vi "SRT-2014-Controls-Basic.vi"() -> ()   [LabVIEW 2013]
uses:
  <vilib>/DAQmx/write.llb/DAQmx Write (Digital Bool 1Line 1Point).vi
  <vilib>/DAQmx/miscellaneous.llb/DAQmx Fill In Error Info.vi
panel:
  out "Ignition":bool
  in  "Ignite":bool
  out "NO2 Venting":bool
  out "NO2 Filling":bool
  in  "Emergency Stop":bool
  in  "Disconnected":bool
  in  "Done W/ NO2":bool
  in  "NO2 QD":bool
  in  "NO2 Vent":bool
  in  "NO2 Fill":bool
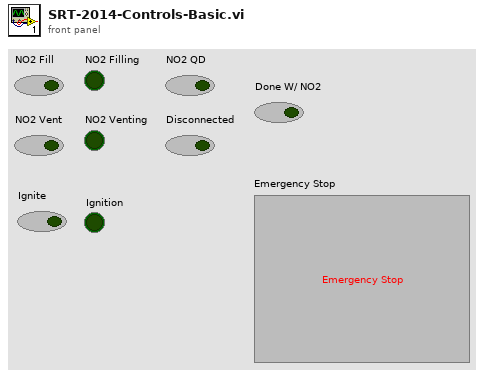
[diagram p1: front panel]
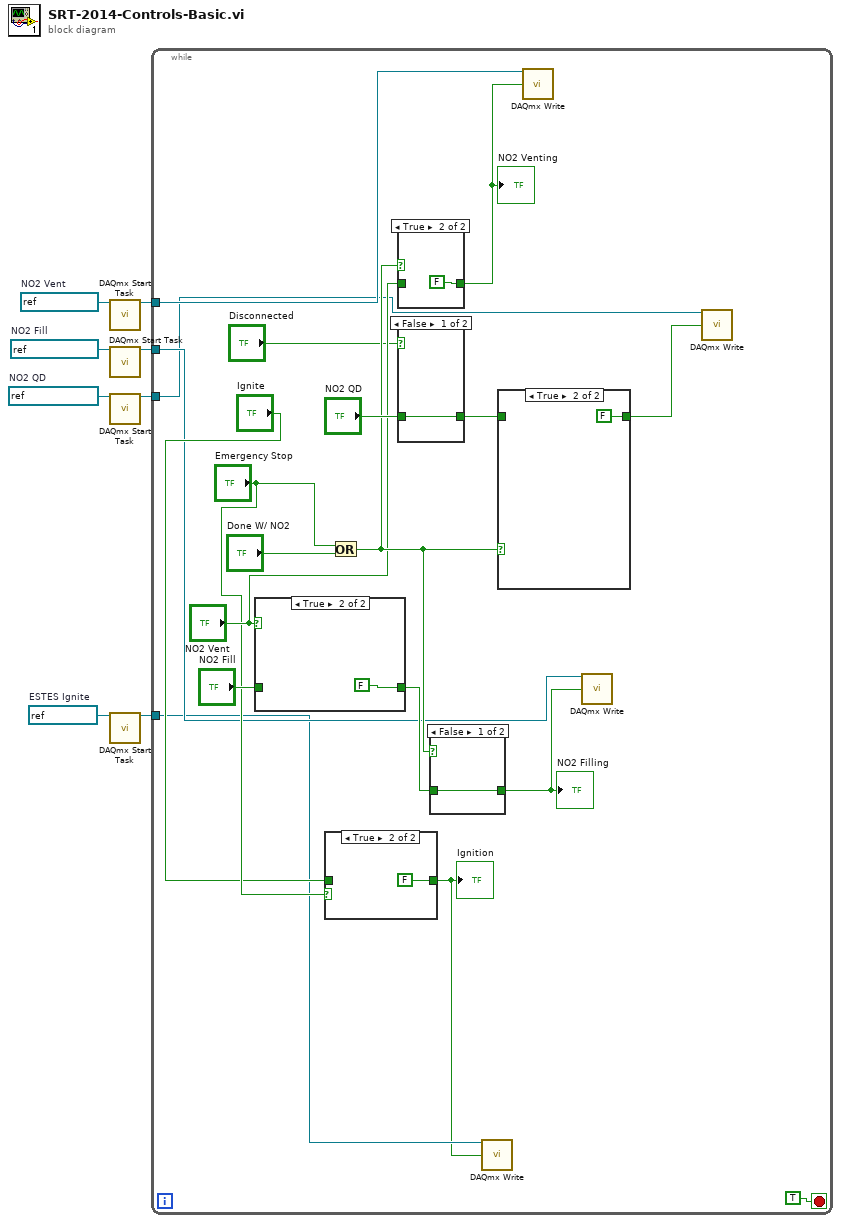
[diagram p0: block diagram]
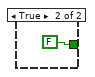
[diagram p4: hidden frame]
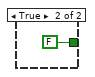
[diagram p6: hidden frame]
diagram:
  w2 = refnum<k21> "2_3"  # ESTES Ignite
  w6 = refnum<k21> "1_0"  # NO2 Fill
  w4 = refnum<k21> "1_2"  # NO2 QD
  w8 = refnum<k21> "1_1"  # NO2 Vent
  n1 = call <vilib>:"DAQmx Start Task.vi"("task/channels in"=w8) -> ("task out"=w7:refnum<k21>)  [unwired: 13 in, 1 out]
  n2 = call <vilib>:"DAQmx Start Task.vi"("task/channels in"=w6) -> ("task out"=w5:refnum<k21>)  [unwired: 13 in, 1 out]
  n3 = call <vilib>:"DAQmx Start Task.vi"("task/channels in"=w4) -> ("task out"=w3:refnum<k21>)  [unwired: 13 in, 1 out]
  n4 = call <vilib>:"DAQmx Start Task.vi"("task/channels in"=w2) -> ("task out"=w1:refnum<k21>)  [unwired: 13 in, 1 out]
  n5 = while {
    tunnel: w7 -> [w16]
    tunnel: w5 -> [w14]
    tunnel: w3 -> [w12]
    tunnel: w1 -> [w10]
    stop <- TRUE stop-if-true
    n6 = case shown="True" "NO2 Vent" {
      tunnel: "NO2 Fill" -> [w38 _]
      tunnel: [w38 FALSE] -> w25
      frame False {
      }
      frame True {
      }
    }
    n7 = case shown="True" "Emergency Stop" {
      tunnel: [w28 FALSE] -> w9
      tunnel: "Ignite" -> [w28 _]
      frame False {
      }
      frame True {
      }
    }
    "Ignition" <- w9
    n8 = Or(x="Emergency Stop", y="Done W/ NO2") -> (x .or. y?=w22:bool)
    n9 = case shown="True" w22 {
      tunnel: [w34 FALSE] -> w15
      tunnel: "NO2 Vent" -> [w34 _]
      frame False {
      }
      frame True {
      }
    }
    "NO2 Venting" <- w15
    n10 = case shown="False" "Disconnected" {
      tunnel: "NO2 QD" -> [w36 _]
      tunnel: [w36 FALSE] -> w24
      frame False {
      }
      frame True {
      }
    }
    n11 = case shown="False" w22 {
      tunnel: w25 -> [w32 _]
      tunnel: [w32 FALSE] -> w13
      frame False {
      }
      frame True {
      }
    }
    "NO2 Filling" <- w13
    n12 = call-poly <vilib>:"DAQmx Write.vi"("task/channels in"=w10, "data"=w9) -> ()  [unwired: 11 in, 3 out]
    n13 = case shown="True" w22 {
      tunnel: w24 -> [w30 _]
      tunnel: [w30 FALSE] -> w11
      frame False {
      }
      frame True {
      }
    }
    n14 = call-poly <vilib>:"DAQmx Write.vi"("task/channels in"=w16, "data"=w15) -> ()  [unwired: 11 in, 3 out]
    n15 = call-poly <vilib>:"DAQmx Write.vi"("task/channels in"=w14, "data"=w13) -> ()  [unwired: 11 in, 3 out]
    n16 = call-poly <vilib>:"DAQmx Write.vi"("task/channels in"=w12, "data"=w11) -> ()  [unwired: 11 in, 3 out]
  }
